vi "asyncvistopsfromabort.vi"(11 "channel":T1) -> (3 "other channel out":T1)   [LabVIEW 2020, in "Tests Event MessengerM.lvclass"]
uses:
  Tests Event MessengerM.lvclass
  source/Event MessengerM.lvlib
  source/))Channel.ctl
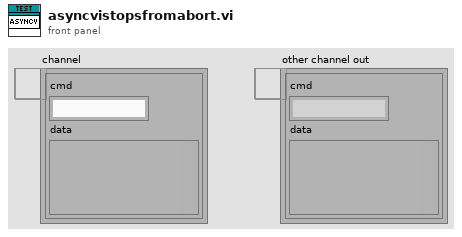
[diagram p1: front panel]
types:
  T1 = typedef "Event MessengerM.lvlib/))Channel.ctl" = refnum<queue>
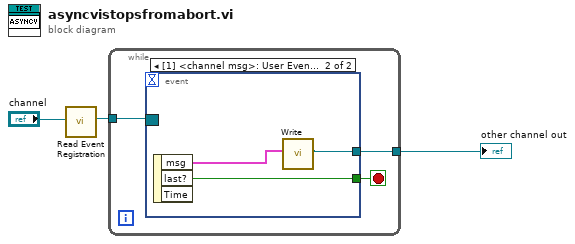
[diagram p0: block diagram]
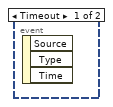
[diagram p2: hidden frame]
diagram:
  n1 = call "Read Event Registration.vi"("channel"="channel") -> ("event registration refnum"=w2:refnum<event-registration>)  [unwired: 10 in]
  n2 = while {
    tunnel: w2 -> [w6]
    tunnel: [w4] -> w1
    stop <- w5 stop-if-true
    n3 = event shown="[1] <channel msg>: User Event" {
      selector: w6 -> [_ _]
      dyn-events: _ -> [_ _]
      timeout: _ -> [_ _]
      tunnel: [_ w9] -> w5
      tunnel: [_ w7] -> w4
      event Timeout {
        n4 = event-data() -> ()  [unwired: 1 in, 3 out]
      }
      event User Event {
        n5 = event-data() -> ("msg"=w8:cluster{"cmd":string, "data":variant}, "last?"=w9:bool)  [unwired: 1 in, 1 out]
        n6 = call "Write.vi"("element"=w8) -> ("channel"=w7:T1)  [unwired: 9 in, 1 out]
      }
    }
  }
  "other channel out" <- w1
